vi "FTW-CodeGen-GetHelp.vi"(0 "State In":T4, 5 "XRef":refnum<vi>, 7 "Point":cluster{"Horizontal":i32, "Vertical":i32}) -> (4 "Standard Help Info":T3, 6 "Detailed Help Info":T2, 8 "Subitem Help Info":T1, 10 "Use Detailed Help?":bool, 15 "Use Subitem Help?":bool)   [LabVIEW 2015, in "FTW-dotNet-MySQL-Fetch.xnode"]
uses:
  FTW-dotNet-MySQL-Fetch.xnode
  FTW-CodeGen-State.ctl
panel:
  # "Inputs"
  # "Outputs"
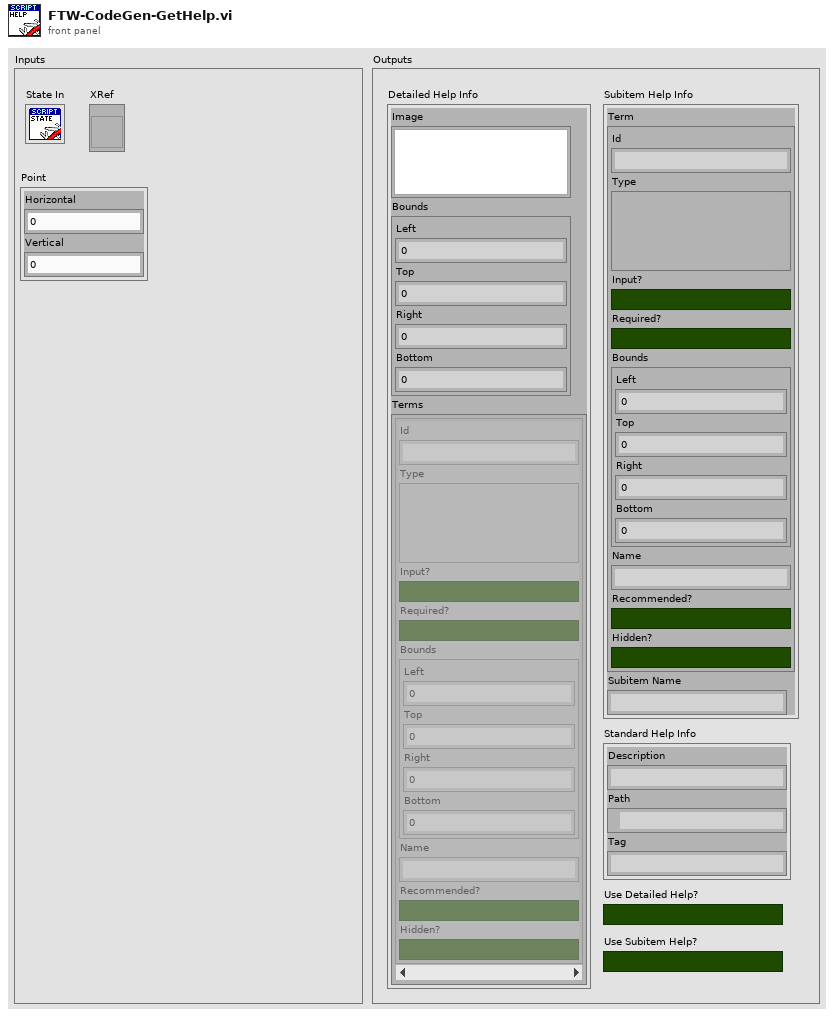
[diagram p1: front panel]
types:
  T1 = cluster{"Term":cluster{"Id":string, "Type":variant, "Input?":bool, "Required?":bool, "Bounds":cluster{"Left":i32, "Top":i32, "Right":i32, "Bottom":i32}, "Name":string, "Recommended?":bool, "Hidden?":bool}, "Subitem Name":string}
  T2 = cluster{"Image":picture, "Bounds":cluster{"Left":i32, "Top":i32, "Right":i32, "Bottom":i32}, "Terms":cluster{"Id":string, "Type":variant, "Input?":bool, "Required?":bool, "Bounds":cluster{"Left":i32, "Top":i32, "Right":i32, "Bottom":i32}, "Name":string, "Recommended?":bool, "Hidden?":bool}[]}
  T3 = cluster{"Description":string, "Path":path, "Tag":string}
  T4 = typedef "FTW-dotNet-MySQL-Fetch.xnode/FTW-CodeGen-State.ctl" = cluster{"Dummy":string}
  T5 = cluster{"Id":string, "Type":variant, "Input?":bool, "Required?":bool, "Bounds":cluster{"Left":i32, "Top":i32, "Right":i32, "Bottom":i32}, "Name":string, "Recommended?":bool, "Hidden?":bool}
  T6 = cluster{"Name":string, "Id":string, "Type":variant, "Bounds":cluster{"Left":i32, "Top":i32, "Right":i32, "Bottom":i32}, "Input?":bool, "Required?":bool, "Recommended?":bool, "Adaptive?":bool, "Hidden?":bool, "Direction":enum32{"Auto", "Up", "Down", "Left", "Right", "Center"}, "Break Wire?":bool, "English Name":string}[]
  T7 = cluster{"Left":i32, "Top":i32, "Right":i32, "Bottom":i32}
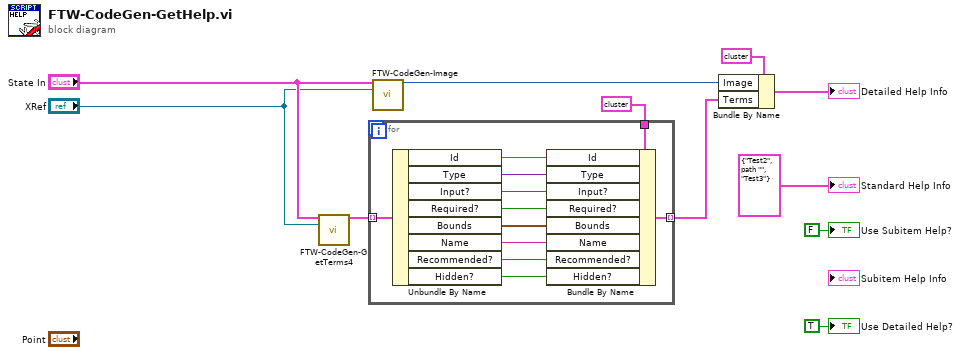
[diagram p0: block diagram]
diagram:
  n1 = call "FTW-CodeGen-GetTerms4.vi"("State In"="State In", "XRef"="XRef") -> ("Terms"=w5:T6)  [unwired: 13 in]
  n2 = for {
    tunnel: [w21] -> w7 mode=indexing
    tunnel: T5 {"Id"="", "Type"=variant, "Input?"=FALSE, "Required?"=FALSE, "Bounds"={"Left"=0, "Top"=0, "Right"=0, "Bottom"=0}, "Name"="", "Recommended?"=FALSE, "Hidden?"=FALSE} ("Term") -> [w22]
    tunnel: w5 -> [w20] mode=indexing
    n3 = Unbundle By Name(w20) -> ("Id"=w19:string, "Type"=w18:variant, "Input?"=w17:bool, "Required?"=w16:bool, "Bounds"=w15:T7, "Name"=w14:string, "Recommended?"=w13:bool, "Hidden?"=w12:bool)
    n4 = Bundle By Name(cluster=w22, "Id"=w19, "Type"=w18, "Input?"=w17, "Required?"=w16, "Bounds"=w15, "Name"=w14, "Recommended?"=w13, "Hidden?"=w12) -> (w21:T5)
  }
  n5 = call "FTW-CodeGen-Image.vi"("State In"="State In", "XRef"="XRef") -> ("Image"=w8:picture)  [unwired: 13 in]
  n6 = Bundle By Name(cluster=T2 {"Image"=bytes[0], "Bounds"={"Left"=0, "Top"=0, "Right"=0, "Bottom"=0}, "Terms"=[]} ("Detailed Help Info"), "Image"=w8, "Terms"=w7) -> (→"Detailed Help Info":T2)
  "Standard Help Info" <- T3 {"Description"="Test2", "Path"=path "", "Tag"="Test3"} ("Standard Help Info")
  "Use Detailed Help?" <- TRUE ("Use Detailed Help?")
  "Use Subitem Help?" <- FALSE ("Use Subitem Help?")
